vi "PrgDisplay.vi"(8 "error in (no error)":errorcluster, 10 "PRG in":refnum<class "Cycle.lvclass">[](array[class]), 11 "PRG List Refnum":refnum<vi>) -> (0 "error out":errorcluster)   [LabVIEW 2012, in "StimulCtrls.lvlib"]
uses:
  StimulCtrls.lvlib
  CYL/Cycle.lvclass
panel:
  in  "Program List":i32(listbox)
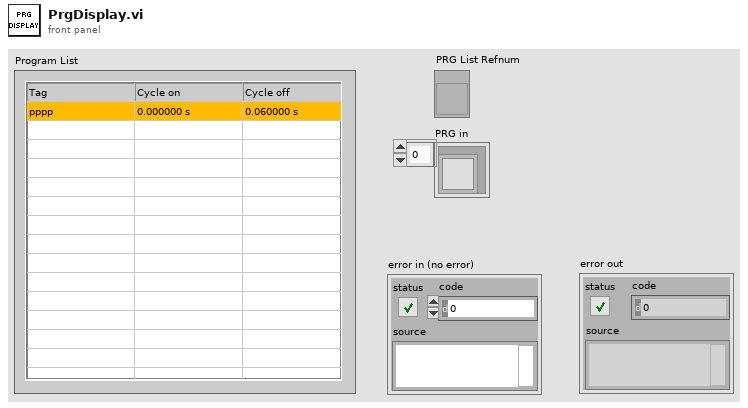
[diagram p1: front panel]
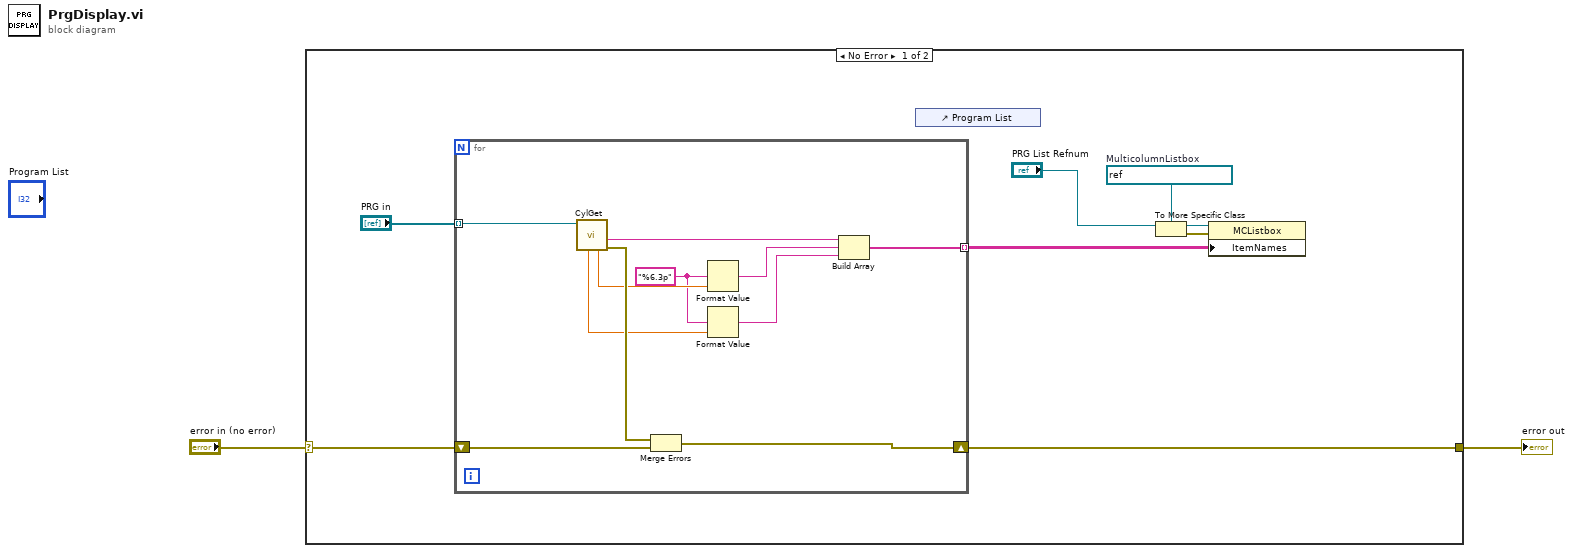
[diagram p0: block diagram]
diagram:
  n1 = case shown="No Error" "error in (no error)" {
    selector: "error in (no error)" -> [w6 w22]
    tunnel: [w4 w22] -> w1
    frame No Error {
      w8 = refnum<vi> refnum  # MulticolumnListbox
      n2 = for {
        tunnel: "PRG in" -> [w21] mode=indexing
        shift-right: [w18] -> w4
        shift-left: w6 -> [w20]
        tunnel: [w12] -> w5 mode=indexing
        w11 = "%6.3p" ("format string")
        n3 = call-dynamic "CylGet.vi"("Cycle in"=w21) -> ("error out"=w19:errorcluster, "Tag"=w17:string, "Cycle on"=w16:dbl[unit], "Cycle off"=w14:dbl[unit])  [unwired: 5 in, 2 out]
        n4 = Merge Errors(w19, w20) -> (w18:errorcluster)
        n5 = Format Value(format string=w11, value (0)=w16) -> (output string=w15:string)  [unwired: 1 in]
        n6 = Format Value(format string=w11, value (0)=w14) -> (output string=w13:string)  [unwired: 1 in]
        n7 = Build Array(w17, w15, w13) -> (w12:string[])
      }
      n8 = control-ref of="Program List"() -> ()  [unwired: 1 out]
      n9 = To More Specific Class(target class=w8, reference="PRG List Refnum") -> (specific class reference=w10:refnum<vi>, error out=w9:errorcluster)  [unwired: 1 in]
      n10 = property class="MCListbox"(reference=w10, error in=w9, "ItemNames"=w5) -> ()  [unwired: 2 out]
    }
    frame Error {
    }
  }
  "error out" <- w1
